vi "Balance.vi"(2 "Segway Mode?":bool, 3 "Pitch Angle":dbl, 4 "Right Axis":dbl, 5 "Left Axis":dbl) -> (0 "Right Axis":dbl, 1 "Left Axis":dbl)   [LabVIEW 2015]
panel:
  in  "PID Gains":cluster{"Kp":dbl, "Ki":dbl, "Kd":dbl}={"Kp"=0.05, "Ki"=0.0, "Kd"=0.0}
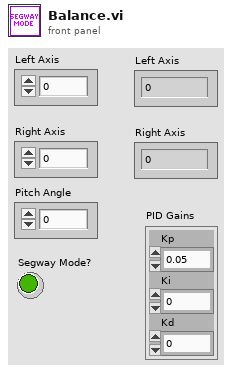
[diagram p1: front panel]
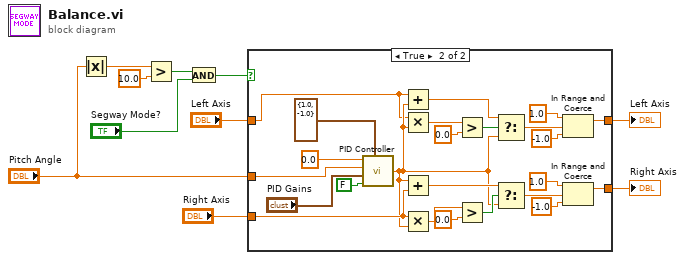
[diagram p0: block diagram]
diagram:
  n1 = Absolute Value(x="Pitch Angle") -> (abs(x)=w6:dbl)
  n2 = Greater?(x=w6, y=10.0 ("Pitch Angle")) -> (0:w9:bool)
  n3 = And(x=w9, y="Segway Mode?") -> (x .and. y?=w7:bool)
  n4 = case shown="True" w7 {
    tunnel: "Left Axis" -> [w11 w14]
    tunnel: "Right Axis" -> [w12 w27]
    tunnel: [w12 w25] -> w3
    tunnel: [w11 w13] -> w2
    tunnel: "Pitch Angle" -> [_ w33]
    frame False {
    }
    frame True {
      n5 = call "PID Controller.vi"("setpoint"=0.0, "process variable"=w33, "PID Gains"="PID Gains", "Reinitialize Integral"=FALSE, "Constrain"=cluster{"Max Control":dbl, "Min Control":dbl} {"Max Control"=1.0, "Min Control"=-1.0}) -> ("Control Signal"=w15:dbl)
      n6 = Add(x=w14, y=w15) -> (x+y=w18:dbl)
      n7 = Multiply(x=w14, y=w15) -> (x*y=w21:dbl)
      n8 = Add(x=w15, y=w27) -> (x+y=w26:dbl)
      n9 = Multiply(x=w27, y=w15) -> (x*y=w30:dbl)
      n10 = Greater?(x=w21, y=0.0) -> (0:w19:bool)
      n11 = Greater?(x=w30, y=0.0) -> (0:w28:bool)
      n12 = Select(t=w18, s=w19, f=w15) -> (s? t:f=w22:dbl)
      n13 = Select(t=w26, s=w28, f=w15) -> (s? t:f=w31:dbl)
      n14 = In Range and Coerce(upper limit=1.0, x=w22, lower limit=-1.0) -> (coerced(x)=w13:dbl)  [unwired: 1 out]
      n15 = In Range and Coerce(upper limit=1.0, x=w31, lower limit=-1.0) -> (coerced(x)=w25:dbl)  [unwired: 1 out]
    }
  }
  "Left Axis" <- w2
  "Right Axis" <- w3
